vi "RT_REG_PIReg.vi"(9 "Reg_Param":T2={"Byp"=FALSE, "En"=FALSE, "Reinit"=FALSE, "Hold"=FALSE, "Preset"=FALSE, "Kp"=1.0, "Ki"=1.0, "Freq (Hz)"=1.0, "Reinit_Val"=0.0, "Out_Rg_HiLim"=0.0, "Out_Rg_LowLim"=0.0, "Byp_Ref"=0.0, "Preset_Ref"=0.0} {"Preset_Ref" format="%.2f"; "Byp_Ref" format="%.2f"; "Out_Rg_LowLim" format="%.3f"; "Out_Rg_HiLim" format="%.3f"; "Freq (Hz)" format="%.3f"; "Ki" format="%.3f"; "Kp" format="%.3f"}, 11 "Error (ERR)":sgl format="%.2f") -> (1 "Reg_Sts":T1={"Byp?"=FALSE, "En?"=FALSE, "Reinit?"=FALSE, "Hold?"=FALSE, "OutOfRg?"=FALSE, "Prop_Out"=1.0, "Int_Out"=1.0, "Int_Acc_Out"=1.0, "Int_Acc_Last"=1.0} {"Int_Acc_Last" format="%.3f"; "Int_Acc_Out" format="%.3f"; "Int_Out" format="%.3f"; "Prop_Out" format="%.3f"}, 3 "Out (CV)":sgl format="%.2f")   [LabVIEW 2024]
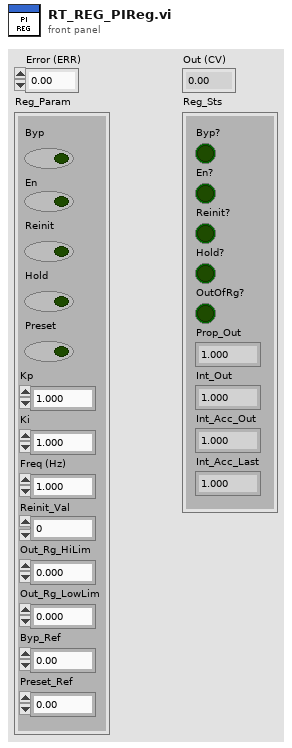
[diagram p1: front panel]
types:
  T1 = cluster{"Byp?":bool, "En?":bool, "Reinit?":bool, "Hold?":bool, "OutOfRg?":bool, "Prop_Out":sgl, "Int_Out":sgl, "Int_Acc_Out":sgl, "Int_Acc_Last":sgl}
  T2 = cluster{"Byp":bool, "En":bool, "Reinit":bool, "Hold":bool, "Preset":bool, "Kp":sgl, "Ki":sgl, "Freq (Hz)":sgl, "Reinit_Val":sgl, "Out_Rg_HiLim":sgl, "Out_Rg_LowLim":sgl, "Byp_Ref":sgl, "Preset_Ref":sgl}
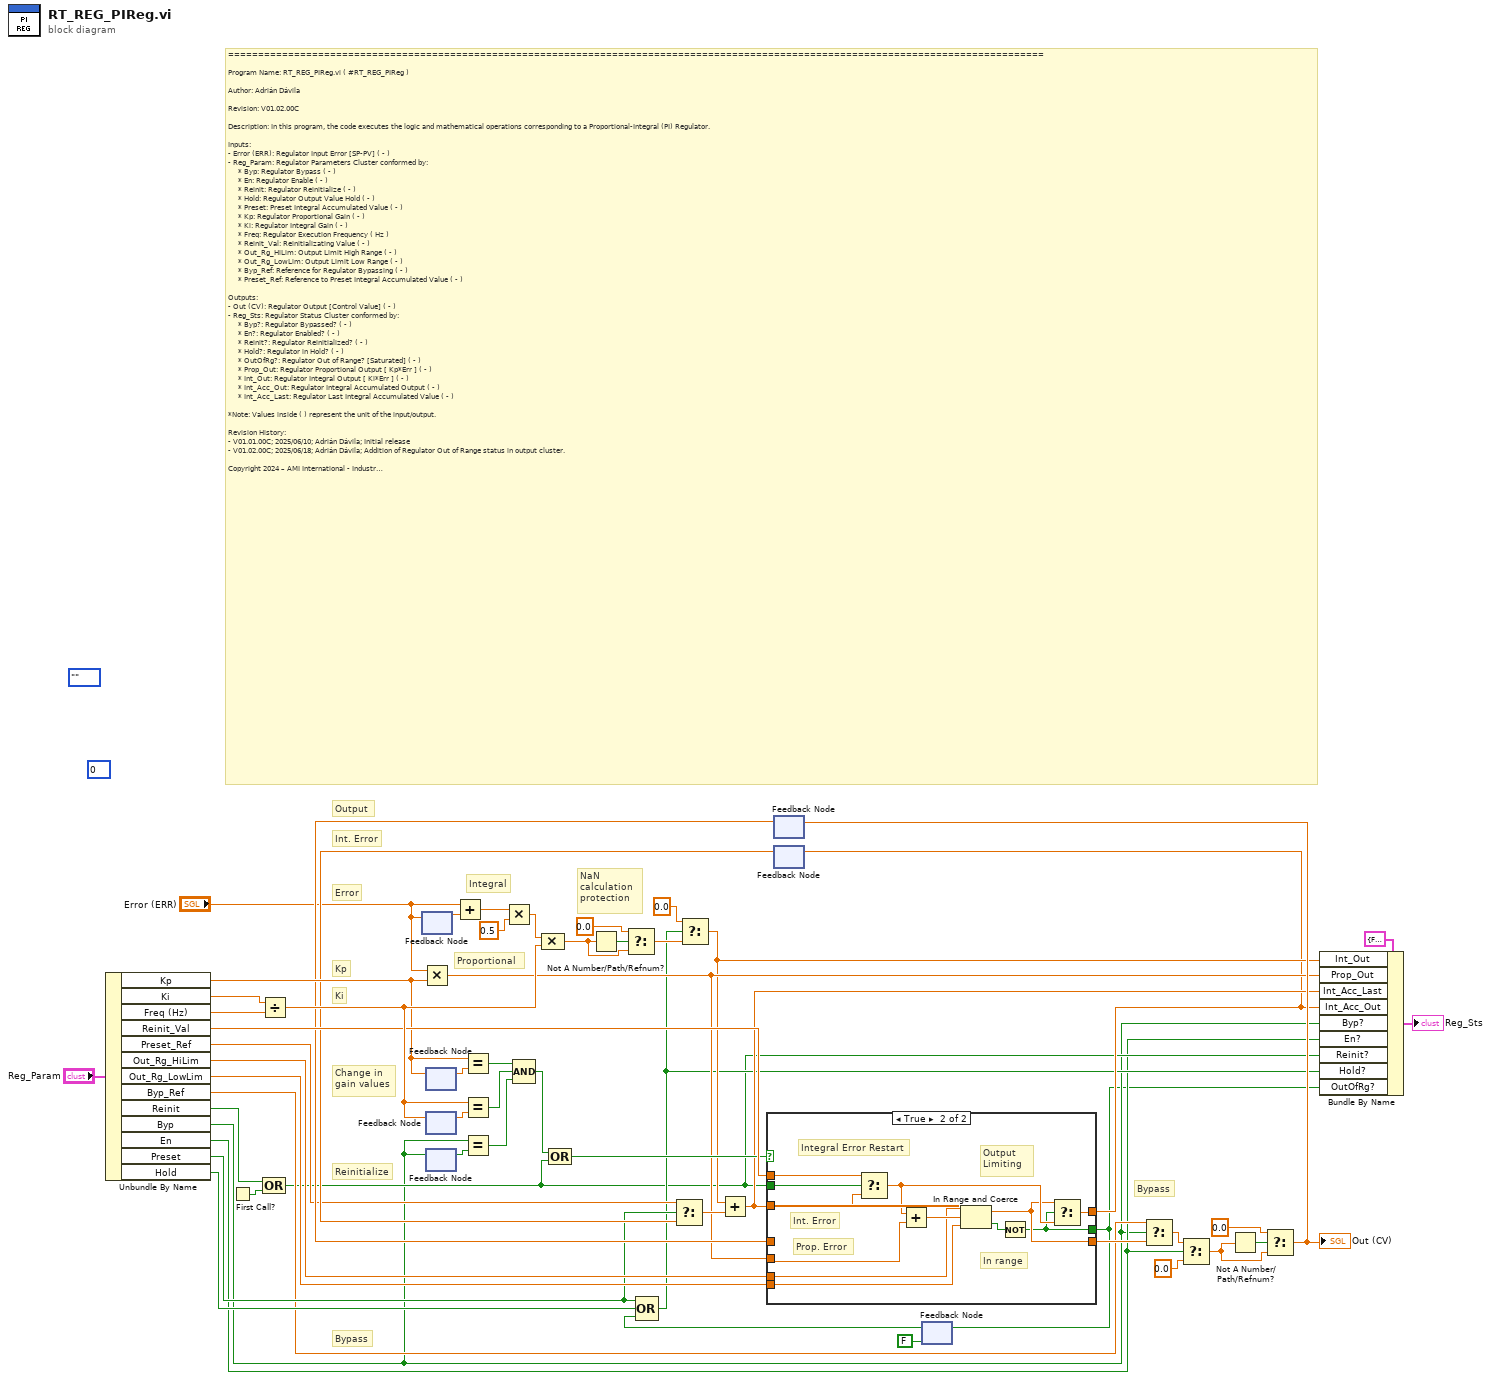
[diagram p0: block diagram]
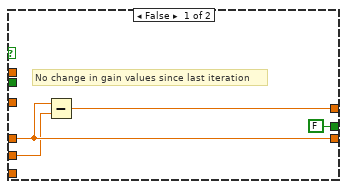
[diagram p2: hidden frame]
diagram:
  (unwired) u16 0 items=[""]
  (unwired) enum16{""}.""
  # "Bypass"
  # "Change in\ngain values"
  # "Int. Error"
  # "Output"
  # "Reinitialize"
  # "Ki"
  # "Kp"
  # "Bypass"
  # "Error"
  # "Proportional"
  # "Integral"
  # "NaN calculation protection"
  # "========================================================================================================================================\n\nProgram Name: RT_REG_PIReg.vi ( #RT_REG_PIReg )\n\nAuthor: Adrián Dávila\n\nRevision: V01.02.00C\n\nDescription: In this program, the code executes the logic and mathematical operations corresponding to a Proportional-Integral (PI) Regulator. \n\nInputs:\n- Error (ERR): Regulator Input Error [SP-PV] ( - )\n- Reg_Param: Regulator Parameters Cluster conformed by:\n     * Byp: Regulator Bypass ( - )\n     * En: Regulator Enable ( - )\n     * Reinit: Regulator Reinitialize ( - )\n     * Hold: Regulator Output Value Hold ( - )\n     * Preset: Preset Integral Accumulated Value ( - )\n     * Kp: Regulator Proportional Gain ( - )\n     * Ki: Regulator Integral Gain ( - )\n     * Freq: Regulator Execution Frequency ( Hz )\n     * Reinit_Val: Reinitializating Value ( - )\n     * Out_Rg_HiLim: Output Limit High Range ( - )\n     * Out_Rg_LowLim: Output Limit Low Range ( - )\n     * Byp_Ref: Reference for Regulator Bypassing ( - )\n     * Preset_Ref: Reference to Preset Integral Accumulated Value ( - )\n\nOutputs:\n- Out (CV): Regulator Output [Control Value] ( - )\n- Reg_Sts: Regulator Status Cluster conformed by:\n     * Byp?: Regulator Bypassed? ( - )\n     * En?: Regulator Enabled? ( - )\n     * Reinit?: Regulator Reinitialized? ( - )\n     * Hold?: Regulator in Hold? ( - )\n     * OutOfRg?: Regulator Out of Range? [Saturated] ( - )\n     * Prop_Out: Regulator Proportional Output [ Kp*Err ] ( - )\n     * Int_Out: Regulator Integral Output [ Ki*Err ] ( - )\n     * Int_Acc_Out: Regulator Integral Accumulated Output ( - )\n     * Int_Acc_Last: Regulator Last Integral Accumulated Value ( - )\n\n*Note: Values inside ( ) represent the unit of the input/output.\n \nRevision History: \n- V01.01.00C; 2025/06/10; Adrián Dávila; Initial release\n- V01.02.00C; 2025/06/18; Adrián Dávila; Addition of Regulator Out of Range status in output cluster.\n\nCopyright 2024 – AMI International - Industrial Solutions\n\n========================================================================================================================================"
  n1 = Unbundle By Name("Reg_Param") -> ("Kp"=w48:sgl, "Ki"=w49:sgl, "Freq (Hz)"=w50:sgl, "Reinit_Val"=w52:sgl, "Preset_Ref"=w12:sgl, "Out_Rg_HiLim"=w18:sgl, "Out_Rg_LowLim"=w19:sgl, "Byp_Ref"=w14:sgl, "Reinit"=w51:bool, "Byp"=w4:bool, "En"=w5:bool, "Preset"=w17:bool, "Hold"=w15:bool)
  n2 = First Call?() -> (First Call?: T/F=w55:bool)
  n3 = Divide(x=w49, y=w50) -> (x/y=w54:sgl)
  n4 = Compound Arithmetic op=OR(w51, w55) -> (w6:bool)
  n5 = feedback #1() -> (w38:sgl)  [unwired: 1 in]
  n6 = feedback-in #1("Error (ERR)") -> ()
  n7 = Multiply(x="Error (ERR)", y=w48) -> (x*y=w11:sgl)
  n8 = feedback #2() -> (w36:sgl)  [unwired: 1 in]
  n9 = feedback-in #2(w48) -> ()
  n10 = feedback #3() -> (w37:sgl)  [unwired: 1 in]
  n11 = feedback-in #3(w54) -> ()
  n12 = feedback #4() -> (w35:bool)  [unwired: 1 in]
  n13 = feedback-in #4(w4) -> ()
  n14 = Add(x="Error (ERR)", y=w38) -> (x+y=w43:sgl)
  n15 = Equal?(x=w48, y=w36) -> (x = y?=w47:bool)
  n16 = Equal?(x=w54, y=w37) -> (x = y?=w46:bool)
  n17 = Equal?(x=w4, y=w35) -> (x = y?=w24:bool)
  n18 = Multiply(x=w43, y=sgl 0.5) -> (x*y=w42:sgl)
  n19 = Compound Arithmetic op=AND(w47, w46, w24) -> (w45:bool)
  n20 = Compound Arithmetic op=MULTIPLY(w42, w54) -> (w27:sgl)
  n21 = Compound Arithmetic op=OR(w45, w6) -> (w41:bool)
  n22 = Not A Number/Path/Refnum?(number/path/refnum=w27) -> (NaN/Path/Refnum?=w34:bool)
  n23 = Select(t=sgl 0.0 ("initial condition"), s=w34, f=w27) -> (s? t:f=w26:sgl)
  n24 = feedback #5() -> (w23:sgl)  [unwired: 1 in]
  n25 = feedback #6() -> (w21:sgl)  [unwired: 1 in]
  n26 = Select(t=w12, s=w17, f=w21) -> (s? t:f=w20:sgl)
  n27 = feedback #7(FALSE) -> (w16:bool)
  n28 = Compound Arithmetic op=OR(w17, w15, w16) -> (w7:bool)
  n29 = Select(t=sgl 0.0, s=w7, f=w26) -> (s? t:f=w10:sgl)
  n30 = Add(x=w10, y=w20) -> (x+y=w9:sgl)
  n31 = case shown="True" w41 {
    tunnel: w9 -> [_ w70]
    tunnel: w11 -> [w57 w61]
    tunnel: w23 -> [w59 _]
    tunnel: w6 -> [_ w69]
    tunnel: [w58 w67] -> w8
    tunnel: [w59 w65] -> w25
    tunnel: w52 -> [_ w64]
    tunnel: w18 -> [_ w63]
    tunnel: w19 -> [_ w62]
    tunnel: [FALSE w60] -> w1
    frame False {
      # "No change in gain values since last iteration"
      n32 = Subtract(x=w59, y=w57) -> (x-y=w58:sgl)
    }
    frame True {
      # "In range"
      # "Int. Error"
      # "Prop. Error"
      # "Output Limiting"
      # "Integral Error Restart"
      n33 = Select(t=w64, s=w69, f=w70) -> (s? t:f=w66:sgl)
      n34 = Add(x=w66, y=w61) -> (x+y=w71:sgl)
      n35 = In Range and Coerce(upper limit=w63, x=w71, lower limit=w62) -> (coerced(x)=w65:sgl, In Range?=w68:bool)
      n36 = Not(x=w68) -> (.not. x?=w60:bool)
      n37 = Select(t=w65, s=w60, f=w66) -> (s? t:f=w67:sgl)
    }
  }
  n38 = feedback-in #6(w8) -> ()
  n39 = feedback-in #7(w1) -> ()
  n40 = Select(t=w14, s=w4, f=w25) -> (s? t:f=w30:sgl)
  n41 = Select(t=w30, s=w5, f=sgl 0.0) -> (s? t:f=w29:sgl)
  n42 = Not A Number/Path/Refnum?(number/path/refnum=w29) -> (NaN/Path/Refnum?=w44:bool)
  n43 = Select(t=sgl 0.0 ("initial condition"), s=w44, f=w29) -> (s? t:f=w22:sgl)
  "Out (CV)" <- w22
  n44 = feedback-in #5(w22) -> ()
  n45 = Bundle By Name(cluster=T1 {"Byp?"=FALSE, "En?"=FALSE, "Reinit?"=FALSE, "Hold?"=FALSE, "OutOfRg?"=FALSE, "Prop_Out"=1.0, "Int_Out"=1.0, "Int_Acc_Out"=1.0, "Int_Acc_Last"=1.0} ("Reg_Sts"), "Int_Out"=w10, "Prop_Out"=w11, "Int_Acc_Last"=w9, "Int_Acc_Out"=w8, "Byp?"=w4, "En?"=w5, "Reinit?"=w6, "Hold?"=w7, "OutOfRg?"=w1) -> (→"Reg_Sts":T1)
